vi "15.1.2 FindCordSysbyPattern.vi"() -> ()   [LabVIEW 2016]
uses:
  <vilib>/vision/Image Controls.llb/IMAQ Image.ctl
  <vilib>/vision/Image Controls.llb/Vision Info Type2.ctl
  <vilib>/vision/NI_Vision_Development_Module.lvlib
panel:
  out "CordSys":T1 {"Axis Reference" items=["Direct", "Indirect"]; "Angle (deg)" format="%.2f"; "Origin"."Y" format="%.2f"; "Origin"."X" format="%.2f"}
  out "UUT":T2(plugin-control)
  out "Feature":T2(plugin-control)
  in  "Search Rect":T3={"Left"=0, "Top"=0, "Right"=2147483647, "Bottom"=2147483647, "Rotation"=0.0} {"Rotation" format="%.2f"; "Left" scale=0.0..1024.0; "Right" scale=0.0..1024.0}
  in  "Settings":T4={"Algorithm"=2, "Number of Matches Requested"=1, "Minimum Match Score"=800.0, "SubPixel Accuracy"=TRUE, "Rotation Angle Ranges"=[{"Start"=-45.0, "End"=45.0}], "Show Search Area"=FALSE, "Show Result"=TRUE, "Show Feature Found"=TRUE} {"Rotation Angle Ranges"."End" format="%.1f"; "Rotation Angle Ranges"."Start" format="%.1f"; "Minimum Match Score" min=0 max=1000 format="%.2f"; "Number of Matches Requested" min=1; "Algorithm" items=["All", "Low Discrepancy Sampling", "Grayscale Value Pyramid", "Gradients Pyramid"]}
  # "Run VI and check out the Coordinate System found in the UUT"
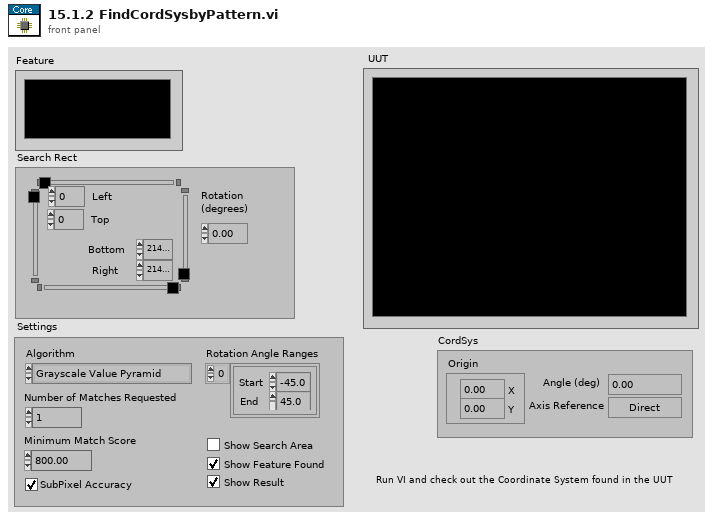
[diagram p1: front panel]
types:
  T1 = cluster{"Origin":cluster{"X":sgl, "Y":sgl}, "Angle (deg)":sgl, "Axis Reference":u32}
  T2 = typedef "IMAQ Image.ctl" = refnum<image>
  T3 = typedef "IMAQ Rectangle" = cluster{"Left":i32, "Top":i32, "Right":i32, "Bottom":i32, "Rotation":dbl}
  T4 = cluster{"Algorithm":i32, "Number of Matches Requested":i32, "Minimum Match Score":sgl, "SubPixel Accuracy":bool, "Rotation Angle Ranges":cluster{"Start":sgl, "End":sgl}[], "Show Search Area":bool, "Show Result":bool, "Show Feature Found":bool}
  T5 = cluster{"Position":cluster{"x":sgl, "y":sgl}, "Angle":sgl, "Scale":sgl, "Score":sgl, "Bounding Box":cluster{"x":sgl, "y":sgl}[]}
  T6 = cluster{"Tmp":T2, "Src":T2, "CordSys":cluster{"Origin":cluster{"X":sgl, "Y":sgl}, "Angle (deg)":sgl, "Axis Reference":u32}, "Search Rect":T3, "element":cluster{"Position":cluster{"x":sgl, "y":sgl}, "Angle":sgl, "Scale":sgl, "Score":sgl, "Bounding Box":cluster{"x":sgl, "y":sgl}[]}, "# Matchs":i32}
  T7 = typedef "Vision Info Type2.ctl" = u32
  T8 = typedef "ROI Descriptor" = cluster{"Global Rectangle":i32[], "Contours":cluster{"ID":enum32{"External", "Internal"}, "Type":u32, "Coordinates":i32[]}[]}
  T9 = cluster{"Number of Matches Requested":i32, "Minimum Match Score":sgl, "Rotation Angle Ranges":cluster{"Start":sgl, "End":sgl}[]}
  T10 = cluster{"Position":cluster{"x":sgl, "y":sgl}, "Angle":sgl, "Scale":sgl, "Score":sgl, "Bounding Box":cluster{"x":sgl, "y":sgl}[]}[]
  T11 = cluster{"Bounding Box[0]":cluster{"x":sgl, "y":sgl}, "Bounding Box[1]":cluster{"x":sgl, "y":sgl}, "Bounding Box[2]":cluster{"x":sgl, "y":sgl}, "Bounding Box[3]":cluster{"x":sgl, "y":sgl}}
  T12 = cluster{"Show Search Area":bool, "Show Feature Found":bool, "Show Result":bool}
  T13 = cluster{cluster{"x":sgl, "y":sgl}, cluster{"x":sgl, "y":sgl}}
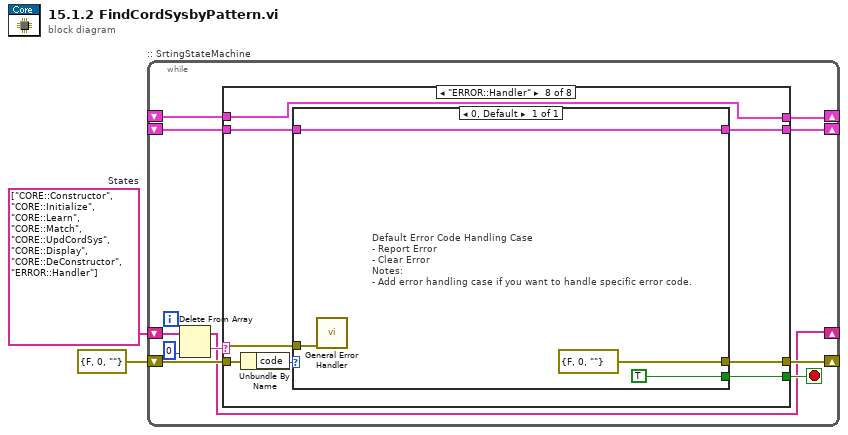
[diagram p0: block diagram]
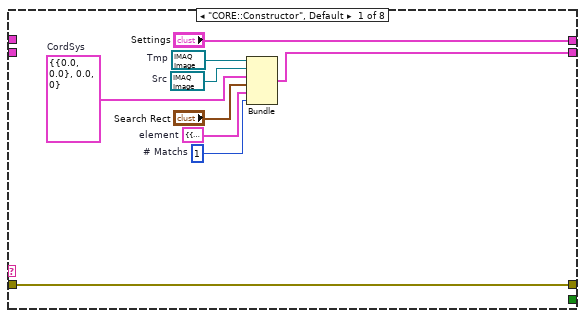
[diagram p2: hidden frame]
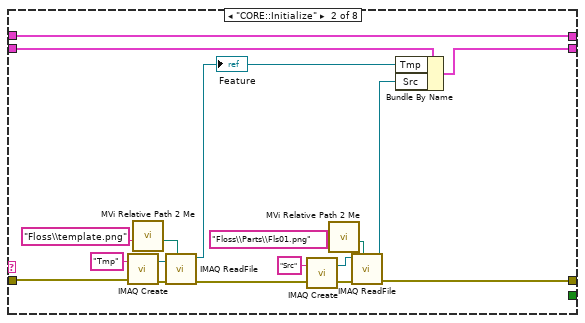
[diagram p3: hidden frame]
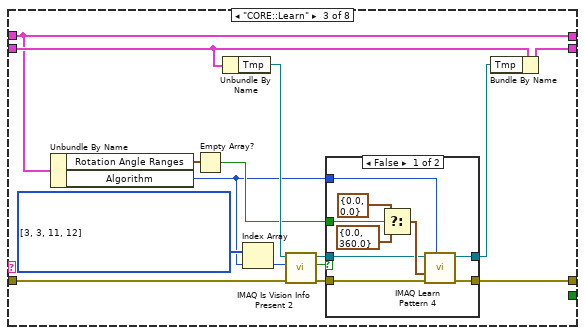
[diagram p4: hidden frame]
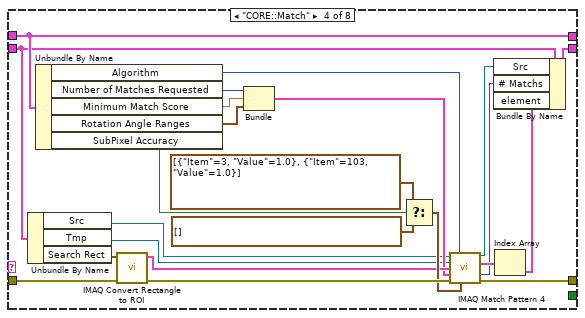
[diagram p6: hidden frame]
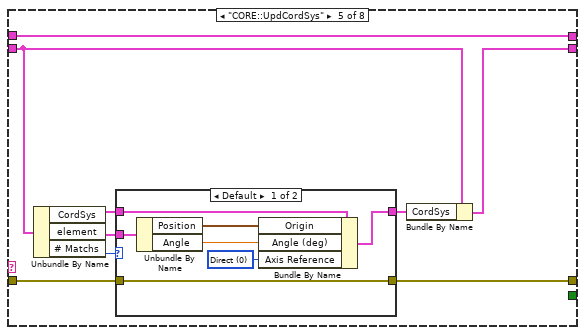
[diagram p7: hidden frame]
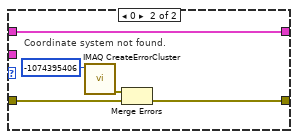
[diagram p8: hidden frame]
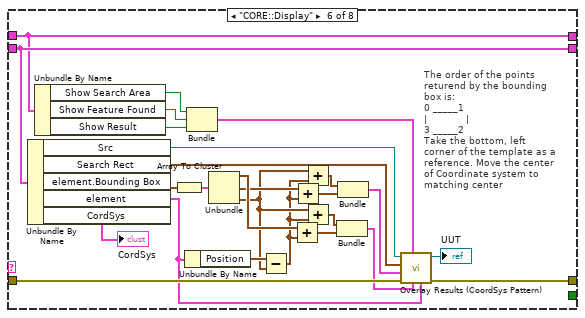
[diagram p9: hidden frame]
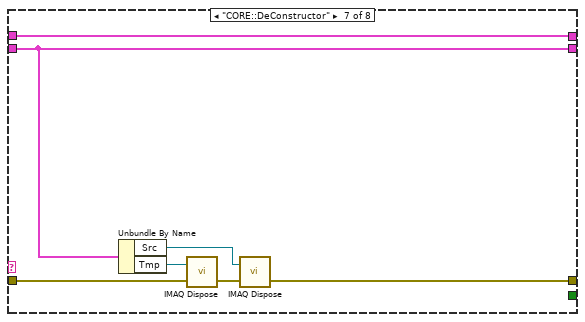
[diagram p10: hidden frame]
diagram:
  w1 = string[] ["CORE::Constructor", "CORE::Initialize", "CORE::Learn", "CORE::Match", "CORE::UpdCordSys", "CORE::Display", "CORE::DeConstructor", "ERROR::Handler"]  # States
  n1 = while ":: SrtingStateMachine" {
    shift-right: [w10] -> _
    shift-left: errorcluster {"status"=FALSE, "code"=0, "source"=""} ("ErrI") -> [w8]
    shift-right: [w12] -> _
    shift-left: _ -> [w11]
    shift-right: [w3] -> _
    shift-left: w1 -> [w9]
    shift-right: [w5] -> _
    shift-left: _ -> [w4]
    stop <- w13 stop-if-true
    n2 = Delete From Array(array=w9, index=0) -> (deleted portion=w7:string, array with subset deleted=w3:string[])  [unwired: 1 in]
    n3 = case shown="\"ERROR::Handler\"" w7 {
      tunnel: [w21 w26 w49 w84 w97 w133 w139 w147] -> w10
      tunnel: [_ _ _ _ _ _ _ w146] -> w13
      tunnel: w8 -> [w21 w34 w53 w86 w98 w132 w143 w145]
      tunnel: [w22 w37 w43 w71 w92 w135 w142 w148] -> w12
      tunnel: w11 -> [_ w38 w44 w72 w93 w135 w142 w149]
      tunnel: ["Settings" w24 w41 w76 w91 w129 w137 w144] -> w5
      tunnel: w4 -> [_ w24 w41 w76 w91 w129 w137 w144]
      frame "CORE::Constructor", Default {
        w14 = T1 {"Origin"={"X"=0.0, "Y"=0.0}, "Angle (deg)"=0.0, "Axis Reference"=0}  # CordSys
        w15 = 1  # # Matchs
        w16 = T5 {"Position"={"x"=0.0, "y"=0.0}, "Angle"=0.0, "Scale"=0.0, "Score"=0.0, "Bounding Box"=[]}  # element
        w19 = T2 refnum  # Src
        w20 = T2 refnum  # Tmp
        n4 = Bundle("Tmp"=w20, "Src"=w19, "CordSys"=w14, "Search Rect"="Search Rect", "element"=w16, "# Matchs"=w15) -> (w22:T6)  [unwired: 1 in]
      }
      frame "CORE::Initialize" {
        n5 = call "IMAQ Create"("Image Name"="Tmp", "error in (no error)"=w34) -> ("Src"=w36:T2, "error out"=w35:errorcluster)  [unwired: 3 in]
        n6 = call "MVi Relative Path 2 Me.vi"("Relative Path"="Floss\\template.png" ("name or relative path")) -> ("Appended Dir"=w28:path)  [unwired: 5 in, 1 out]
        n7 = call "IMAQ ReadFile"("File Path"=w28, "error in (no error)"=w35, "Image"=w36) -> ("error out"=w32:errorcluster, "Image Out"=w23:T2)  [unwired: 4 in, 3 out]
        "Feature" <- w23
        n8 = call "IMAQ Create"("Image Name"="Src", "error in (no error)"=w32) -> ("Src"=w30:T2, "error out"=w31:errorcluster)  [unwired: 3 in]
        n9 = call "MVi Relative Path 2 Me.vi"("Relative Path"="Floss\\Parts\\Fls01.png" ("name or relative path")) -> ("Appended Dir"=w27:path)  [unwired: 5 in, 1 out]
        n10 = call "IMAQ ReadFile"("File Path"=w27, "error in (no error)"=w31, "Image"=w30) -> ("error out"=w26:errorcluster, "Image Out"=w25:T2)  [unwired: 4 in, 3 out]
        n11 = Bundle By Name(cluster=w38, "Tmp"=w23, "Src"=w25) -> (w37:T6)
      }
      frame "CORE::Learn" {
        w55 = T7[] [3, 3, 11, 12] items=["Any", "Calibration", "Overlay", "Grayscale Template", "Color Template", "Geometric Template", "Custom Data", "Golden Template", "Geometric Template 2", "Contour Data", "Camera Model", "Pyramid Grayvalue Template", "Pyramid Gradient Template"]
        n12 = Unbundle By Name(w41) -> ("Rotation Angle Ranges"=w48:cluster{"Start":sgl, "End":sgl}[], "Algorithm"=w46:i32)
        n13 = Empty Array?(array=w48) -> (empty?=w47:bool)
        n14 = Unbundle By Name(w44) -> ("Tmp"=w52:T2)
        n15 = Index Array(array=w55, index=w46) -> (element=w54:T7)
        n16 = call "IMAQ Is Vision Info Present 2"("error in (no error)"=w53, "Vision Info"=w54, "Image"=w52) -> ("error out"=w50:errorcluster, "Present?"=w51:bool, "Image (duplicate)"=w45:T2)  [unwired: 6 out]
        n17 = case shown="False" w51 {
          tunnel: [w64 w65] -> w42
          tunnel: w47 -> [w60 _]
          tunnel: w50 -> [w59 w66]
          tunnel: [w58 w66] -> w49
          tunnel: w46 -> [w57 _]
          tunnel: w45 -> [w56 w65]
          frame False {
            n18 = Select(t=cluster{"Start Angle":sgl, "End Angle":sgl} {"Start Angle"=0.0, "End Angle"=0.0} ("Angle Range"), s=w60, f=cluster{"Start Angle":sgl, "End Angle":sgl} {"Start Angle"=0.0, "End Angle"=360.0} ("Angle Range")) -> (s? t:f=w61:cluster{"Start Angle":sgl, "End Angle":sgl})
            n19 = call "IMAQ Learn Pattern 4"("Algorithm"=w57, "error in (no error)"=w59, "Angle Range"=w61, "Image"=w56) -> ("error out"=w58:errorcluster, "Template Image Out"=w64:T2)  [unwired: 2 in, 4 out]
          }
          frame True {
            # "Already Exist."
          }
        }
        n20 = Bundle By Name(cluster=w44, "Tmp"=w42) -> (w43:T6)
      }
      frame "CORE::Match" {
        n21 = Unbundle By Name(w72) -> ("Src"=w74:T2, "Tmp"=w75:T2, "Search Rect"=w87:T3)
        n22 = Unbundle By Name(w76) -> ("Algorithm"=w69:i32, "Number of Matches Requested"=w80:i32, "Minimum Match Score"=w79:sgl, "Rotation Angle Ranges"=w78:cluster{"Start":sgl, "End":sgl}[], "SubPixel Accuracy"=w83:bool)
        n23 = call "IMAQ Convert Rectangle to ROI"("error in (no error)"=w86, "Rectangle"=w87) -> ("error out"=w85:errorcluster, "ROI Descriptor"=w81:T8)  [unwired: 7 out]
        n24 = Bundle("Number of Matches Requested"=w80, "Minimum Match Score"=w79, "Rotation Angle Ranges"=w78) -> (w77:T9)  [unwired: 1 out]
        n25 = Select(t=cluster{"Item":u16, "Value":dbl}[] [{"Item"=3, "Value"=1.0}, {"Item"=103, "Value"=1.0}] ("Advanced Options"), s=w83, f=cluster{"Item":u16, "Value":dbl}[] [] ("Advanced Options")) -> (s? t:f=w82:cluster{"Item":u16, "Value":dbl}[])
        n26 = call "IMAQ Match Pattern 4"("Image"=w74, "Algorithm"=w69, "Template Image"=w75, "ROI Descriptor"=w81, "Parameters"=w77, "error in (no error)"=w85, "Advanced Options"=w82) -> ("Image (duplicate)"=w70:T2, "Matches (pixel)"=w73:T10, "Number of Matches"=w68:i32, "error out"=w84:errorcluster)  [unwired: 1 in, 4 out]
        n27 = Index Array(array=w73) -> (element=w67:T5)  [unwired: 1 in]
        n28 = Bundle By Name(cluster=w72, "Src"=w70, "# Matchs"=w68, "element"=w67) -> (w71:T6)
      }
      frame "CORE::UpdCordSys" {
        n29 = Unbundle By Name(w93) -> ("CordSys"=w94:T1, "element"=w95:T5, "# Matchs"=w96:i32)
        n30 = case shown="Default" w96 {
          tunnel: [w102 w109] -> w97
          tunnel: w98 -> [w102 w108]
          tunnel: w95 -> [w101 _]
          tunnel: w94 -> [w100 w106]
          tunnel: [w99 w106] -> w90
          frame Default {
            w103 = u32 0 items=["Direct", "Indirect"] ("Axis Reference")
            n31 = Unbundle By Name(w101) -> ("Position"=w104:cluster{"x":sgl, "y":sgl}, "Angle"=w105:sgl)
            n32 = Bundle By Name(cluster=w100, "Origin"=w104, "Angle (deg)"=w105, "Axis Reference"=w103) -> (w99:T1)
          }
          frame 0 {
            # "Coordinate system not found."
            n33 = call "IMAQ CreateErrorCluster"("Error Code"=-1074395406) -> ("error out"=w107:errorcluster)  [unwired: 2 in, 8 out]
            n34 = Merge Errors(w107, w108) -> (w109:errorcluster)
          }
        }
        n35 = Bundle By Name(cluster=w93, "CordSys"=w90) -> (w92:T6)
      }
      frame "CORE::Display" {
        # "The order of the points returend by the bounding box is:\n0 _____1\n|             |\n3 _____2\nTake the bottom, left corner of the template as a reference. Move the center of Coordinate system to matching center"
        n36 = Unbundle By Name(w135) -> ("Src"=w123:T2, "Search Rect"=w124:T3, "element.Bounding Box"=w134:cluster{"x":sgl, "y":sgl}[], "element"=w120:T5, "CordSys"=→"CordSys":T1)
        n37 = Unbundle By Name(w129) -> ("Show Search Area"=w127:bool, "Show Feature Found"=w128:bool, "Show Result"=w126:bool)
        n38 = Array To Cluster(array=w134) -> (cluster=w136:T11)
        n39 = Unbundle By Name(w120) -> ("Position"=w119:cluster{"x":sgl, "y":sgl})
        n40 = Bundle("Show Search Area"=w127, "Show Feature Found"=w128, "Show Result"=w126) -> (w125:T12)  [unwired: 1 out]
        n41 = Unbundle(w136) -> ("Bounding Box[0]"=w118:cluster{"x":sgl, "y":sgl}, "Bounding Box[2]"=w115:cluster{"x":sgl, "y":sgl}, "Bounding Box[3]"=w113:cluster{"x":sgl, "y":sgl})  [unwired: 1 out]
        n42 = Subtract(x=w119, y=w113) -> (x-y=w112:cluster{"x":sgl, "y":sgl})
        n43 = Add(x=w118, y=w112) -> (x+y=w117:cluster{"x":sgl, "y":sgl})
        n44 = Add(x=w115, y=w112) -> (x+y=w114:cluster{"x":sgl, "y":sgl})
        n45 = Add(x=w113, y=w112) -> (x+y=w111:cluster{"x":sgl, "y":sgl})
        n46 = Add(x=w113, y=w112) -> (x+y=w116:cluster{"x":sgl, "y":sgl})
        n47 = Bundle(w116, w117) -> (w131:T13)  [unwired: 1 out]
        n48 = Bundle(w111, w114) -> (w130:T13)  [unwired: 1 out]
        n49 = call <vilib>:"Overlay Results (CoordSys Pattern).vi"("Match"=w120, "Axis 2"=w131, "Setup"=w125, "error in (no error)"=w132, "Axis 1"=w130, "Search Rect"=w124, "Image In"=w123) -> ("error out"=w133:errorcluster, "Image Out"=→"UUT":T2)  [unwired: 3 out]
      }
      frame "CORE::DeConstructor" {
        n50 = Unbundle By Name(w142) -> ("Src"=w138:T2, "Tmp"=w141:T2)
        n51 = call "IMAQ Dispose"("Image"=w141, "error in (no error)"=w143) -> ("error out"=w140:errorcluster)  [unwired: 4 in]
        n52 = call "IMAQ Dispose"("Image"=w138, "error in (no error)"=w140) -> ("error out"=w139:errorcluster)  [unwired: 4 in]
      }
      frame "ERROR::Handler" {
        n53 = Unbundle By Name(w145) -> ("code"=w150:i32)
        n54 = case shown="0, Default" w150 {
          tunnel: [w154] -> w148
          tunnel: w149 -> [w154]
          tunnel: [errorcluster {"status"=FALSE, "code"=0, "source"=""} ("error out")] -> w147
          tunnel: [TRUE] -> w146
          tunnel: w145 -> [w152]
          frame 0, Default {
            # "Default Error Code Handling Case\n- Report Error\n- Clear Error \nNotes:\n- Add error handling case if you want to handle specific error code."
            n55 = call <vilib>:"General Error Handler.vi"("error in (no error)"=w152) -> ()  [unwired: 10 in, 5 out]
          }
        }
      }
    }
  }
